vi "json-demo.vi"() -> ()   [LabVIEW 2017]
panel:
  out "value 2":string
  out "value":i32
  in  "Cluster":cluster{"num":dbl, "str":string}
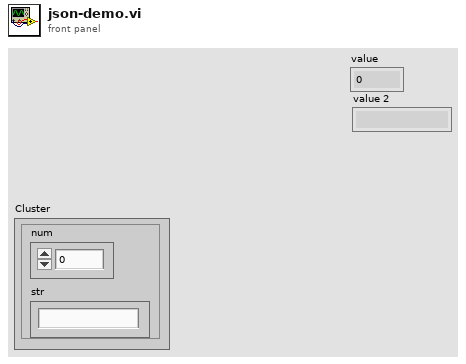
[diagram p1: front panel]
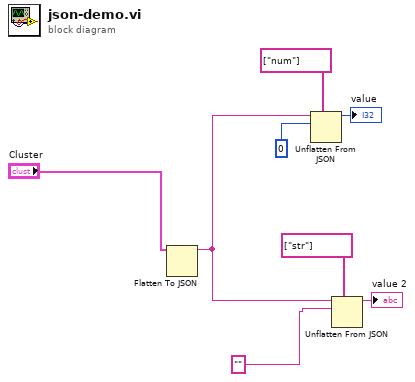
[diagram p0: block diagram]
diagram:
  n1 = Flatten To JSON(anything="Cluster") -> (JSON string=w3:string)  [unwired: 2 in, 1 out]
  n2 = Unflatten From JSON(path=string[] ["num"], JSON string=w3, type and defaults=0) -> (value=→"value":i32)  [unwired: 4 in, 1 out]
  n3 = Unflatten From JSON(path=string[] ["str"], JSON string=w3, type and defaults="") -> (value=→"value 2":string)  [unwired: 4 in, 1 out]
